vi "LuffToSailSuggestion.vi"(6 "OLD Suggested Sail Setpoints":T1 {"MainSailSuggestion" min=0.0 max=1.0; "JibSailSuggestion" min=0.0 max=1.0}, 11 "DegreeOfLuffing":dbl) -> (3 "Suggested Sail Setpoints":T1 {"MainSailSuggestion" min=0.0 max=1.0; "JibSailSuggestion" min=0.0 max=1.0})   [LabVIEW 2012]
doc: "Takes in some measure of the level of luffing in the sail and gives suggestions on how to change the sails to eliminate the luffing and go faster. The simplest case is detecting luffing when on a tack and responding by pulling the sails in a little bit. Check for luffing again after a small delay, and continue \n\nThis algorithm should include some checks to make sure the simple case does not get carried on to ridiculous extremes. For example, we don't want this to find luffing, pull sails in, find luffing, pull sails in, etc. until the sails are locked in - there should be a test to see whether this is driving the sail far out of its wind-lookup position.\n\nTHE SETTINGS COMING OUT OF THIS VI ARE RELATIVE. So if this VI outputs [-0.1, 0.1], it does not mean 'set the main to -0.1 and the jib to 0.1', it means 'adjust the main by 0.1 in and the jib by 0.1 out'.\n\nEric Schneider and Bonnie Ishiguro, Jan. 2014"
uses:
  Data/TypeDefs/Sail Set Suggestions.ctl
panel:
  # "Takes in some measure of the level of luffing in the\nsail and gives suggestions on how to change the\nsails to eliminate the luffing and go faster. The simplest\ncase is detecting luffing when on a tack and responding\nby pulling the sails in a little bit. Check for luffing again\nafter a small delay, and continue \n\nThis algorithm should include some checks to make sure\nthe simple case does not get carried on to ridiculous\nextremes. For example, we don't want this to find luffing,\npull sails in, find luffing, pull sails in, etc. until the sails are\nlocked in - there should be a test to see whether this is\ndriving the sail far out of its wind-lookup position."
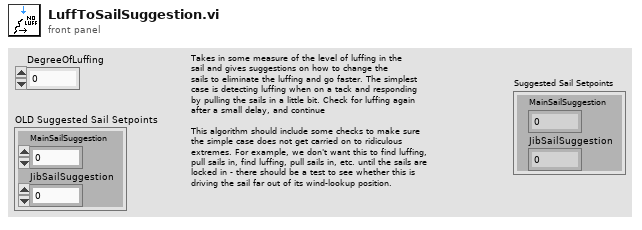
[diagram p1: front panel]
types:
  T1 = typedef "Sail Set Suggestions.ctl" = cluster{"MainSailSuggestion":dbl, "JibSailSuggestion":dbl}
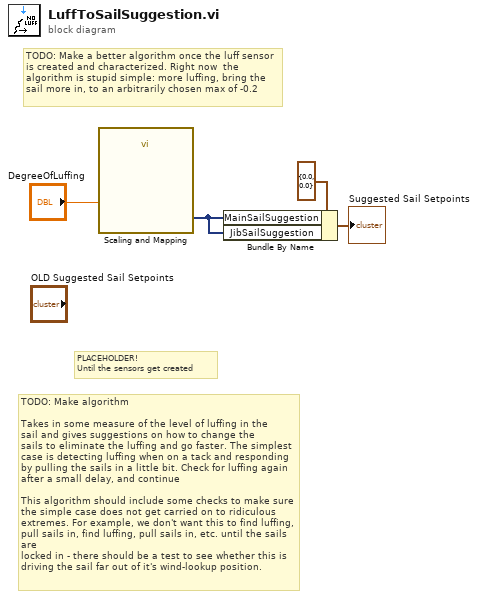
[diagram p0: block diagram]
diagram:
  # "TODO: Make a better algorithm once the luff sensor is created and characterized. Right now  the algorithm is stupid simple: more luffing, bring the sail more in, to an arbitrarily chosen max of -0.2"
  # "PLACEHOLDER!\nUntil the sensors get created"
  # "TODO: Make algorithm\n\nTakes in some measure of the level of luffing in the\nsail and gives suggestions on how to change the\nsails to eliminate the luffing and go faster. The simplest\ncase is detecting luffing when on a tack and responding\nby pulling the sails in a little bit. Check for luffing again\nafter a small delay, and continue \n\nThis algorithm should include some checks to make sure\nthe simple case does not get carried on to ridiculous\nextremes. For example, we don't want this to find luffing,\npull sails in, find luffing, pull sails in, etc. until the sails are\nlocked in - there should be a test to see whether this is\ndriving the sail far out of it's wind-lookup position."
  n1 = call "Scaling and Mapping"("Signals"="DegreeOfLuffing") -> ("Scaled Signals"=w1:dynamicdata)  [unwired: 9 in, 1 out]
  n2 = Bundle By Name(cluster=T1 {"MainSailSuggestion"=0.0, "JibSailSuggestion"=0.0} ("output cluster"), "MainSailSuggestion"=w1, "JibSailSuggestion"=w1) -> (→"Suggested Sail Setpoints":T1)
